vi "xiC - IMAQ - Load_ValChange.vi"(8 "error in (no error)":errorcluster, 11 "Attributes In":T2) -> (0 "error out":errorcluster, 3 "Attributes Out":T2, 4 "State":T1)   [LabVIEW 2015]
uses:
  xiC - IMAQ - States.ctl
  xiC - IMAQ - Attributes.ctl
  C:/GIT/Cameras3.x/Integrations/Labview/xiLib/xiLIB_32bit/xiLIB/xiCamLib/API/x86/xiApi.NET.dll
  xiLIB_32bit/xiLIB/xiCamLib/API/x86/xiApi.NET.dll
  xiC - IMAQ - TreeDisplayType.ctl
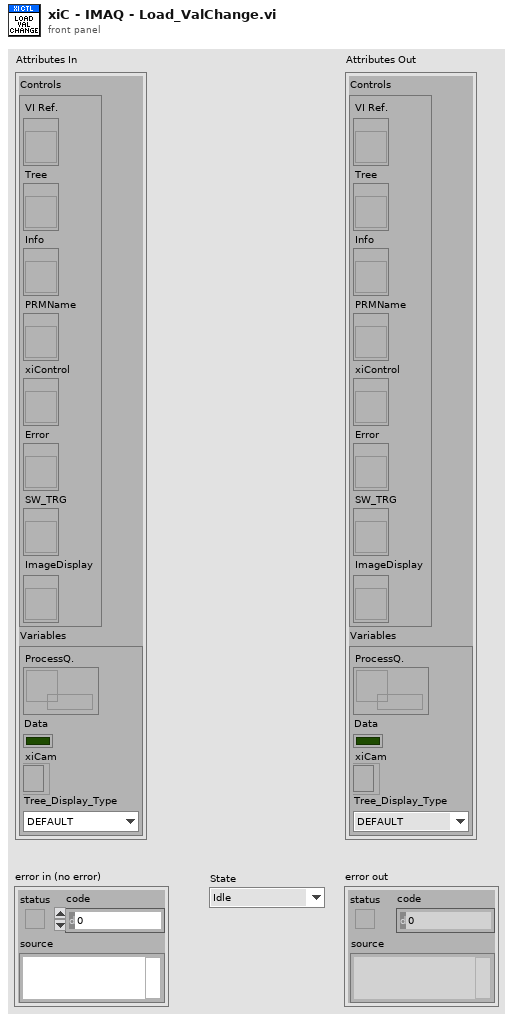
[diagram p1: front panel]
types:
  T1 = typedef "xiC - IMAQ - States.ctl" = enum16{"Idle", "Init", "Exit", "//PRM_UPDATE"}
  T2 = typedef "xiC - IMAQ - Attributes.ctl" = cluster{"Controls":cluster{"VI Ref.":refnum<vi>, "Tree":refnum<vi>, "Info":refnum<vi>, "PRMName":refnum<vi>, "xiControl":refnum<vi>, "Error":refnum<vi>, "SW_TRG":refnum<vi>, "ImageDisplay":refnum<vi>}, "Variables":cluster{"ProcessQ.":refnum<queue>, "Data":bool, "xiCam":refnum<k24>, "Tree_Display_Type":T3}}
  T3 = typedef "xiC - IMAQ - TreeDisplayType.ctl" = enum16{"DEFAULT", "HIDE_MAX_MIN"}
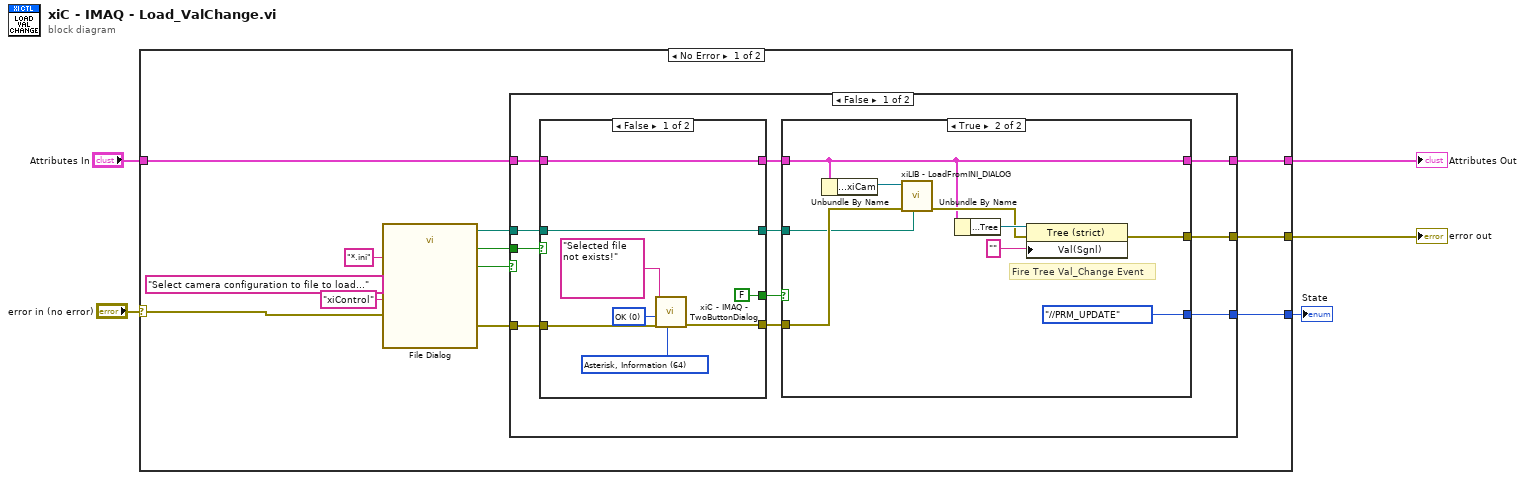
[diagram p0: block diagram]
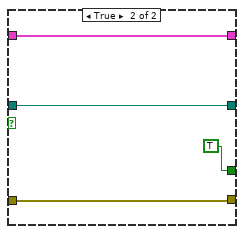
[diagram p3: hidden frame]
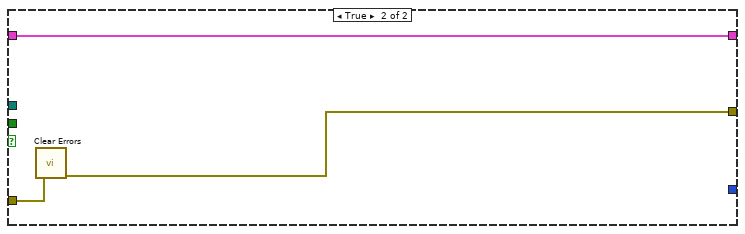
[diagram p4: hidden frame]
diagram:
  n1 = case shown="No Error" "error in (no error)" {
    selector: "error in (no error)" -> [w15 w56]
    tunnel: [w7 w56] -> w4
    tunnel: "Attributes In" -> [w11 w55]
    tunnel: [w8 w55] -> w2
    tunnel: [w6 _] -> w1
    frame No Error {
      n2 = call "File Dialog"("prompt"="Select camera configuration to file to load...", "error in"=w15, "pattern (all files)"="*.ini", "pattern label"="xiControl") -> ("selected path"=w10:path, "exists"=w12:bool, "cancelled"=w14:bool, "error out"=w13:errorcluster)  [unwired: 8 in]
      n3 = case shown="False" w14 {
        tunnel: w13 -> [w27 w54]
        tunnel: w12 -> [w28 _]
        tunnel: w11 -> [w24 w53]
        tunnel: [w22 w53] -> w8
        tunnel: [w21 w52] -> w7
        tunnel: w10 -> [w20 _]
        tunnel: [w18 _] -> w6
        frame False {
          n4 = case shown="False" w28 {
            tunnel: w27 -> [w44 w51]
            tunnel: [FALSE TRUE] -> w26
            tunnel: [w43 w51] -> w25
            tunnel: [w42 w49] -> w23
            tunnel: w24 -> [w42 w49]
            tunnel: w20 -> [w41 w48]
            tunnel: [w41 w48] -> w19
            frame False {
              w46 = 64 items=["None"=0, "Hand, Error, Stop"=16, "Question"=32, "Exclamation, Warning"=48, "Asterisk, Information"=64] ("Icon")
              w45 = 0 items=["OK", "OKCancel", "AbortRetryIgnore", "YesNoCancel", "YesNo", "RetryCancel"] ("Button")
              n5 = call "xiC - IMAQ - TwoButtonDialog.vi"("Icon"=w46, "error in (no error)"=w44, "Button"=w45, "Text"="Selected file not exists!") -> ("error out"=w43:errorcluster)  [unwired: 6 in, 1 out]
            }
            frame True {
            }
          }
          n6 = case shown="True" w26 {
            tunnel: w25 -> [w29 w39]
            tunnel: w23 -> [w30 w33]
            tunnel: [w30 w33] -> w22
            tunnel: [w29 w32] -> w21
            tunnel: w19 -> [_ w38]
            tunnel: [_ xiC_-_IMAQ_-_States."//PRM_UPDATE" ("States")] -> w18
            frame False {
            }
            frame True {
              # "Fire Tree Val_Change Event"
              n7 = Unbundle By Name(w33) -> ("Variables.xiCam"=w37:refnum<k24>)
              n8 = call "xiLIB - LoadFromINI_DIALOG.vi"("IniPath"=w38, "error in (no error)"=w39, "xiCam In"=w37) -> ("error out"=w34:errorcluster)  [unwired: 7 in, 1 out]
              n9 = Unbundle By Name(w33) -> ("Controls.Tree"=w36:refnum<vi>)
              n10 = property class="Tree (strict)"(reference=w36, error in=w34, "Val(Sgnl)"="" ("Value (Signaling)")) -> (error out=w32:errorcluster)  [unwired: 1 out]
            }
          }
        }
        frame True {
          n11 = call <vilib>:"Clear Errors.vi"("error in (no error)"=w54) -> ("error out"=w52:errorcluster)  [unwired: 5 in, 1 out]
        }
      }
    }
    frame Error {
    }
  }
  "error out" <- w4
  "Attributes Out" <- w2
  "State" <- w1
